vi "Relink Package - LV2020.vi"(8 "error in (no error)":errorcluster) -> (0 "error out":errorcluster, 3 "Folder to Relink out":path=path "C:/Users/JonathanGraesser/Downloads/Delacor QMH")   [LabVIEW 2020]
uses:
  3b4289d2-bfe5-4dee-b35d-c917e2b2519d.vi
  44c3ad98-b52a-4573-a8f5-4ecf539941a0.vi
  7ce98f71-275c-4c1e-b900-7d867c156dbc.vi
  c2568c13-bb09-496e-a5a3-529df0c50f32.vi
panel:
  out "report log out":string[](array[string])
  out "Done":bool
  out "all lv items":path[](array[path])
  in  "Folder to relink":string
  out "Saved Items out":T1(array[cluster])
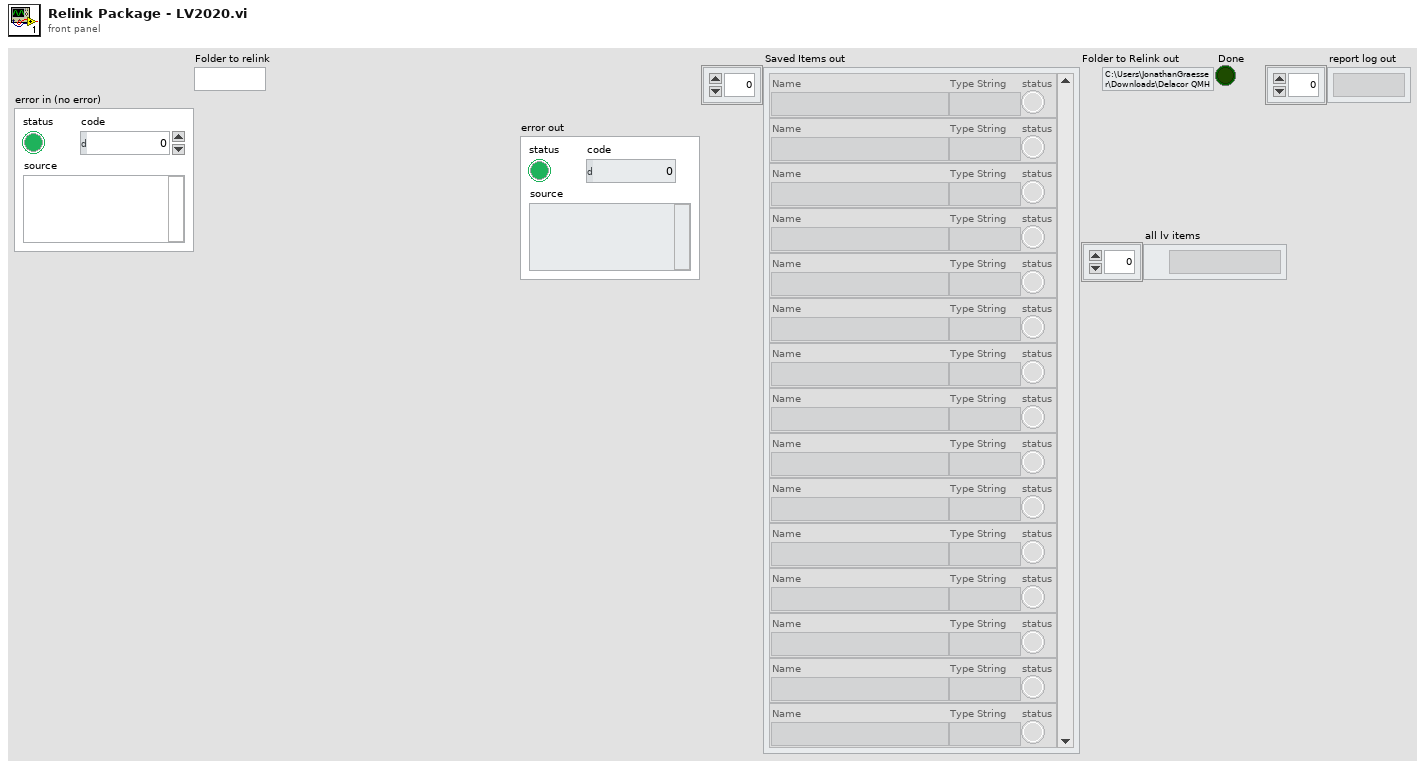
[diagram p1: front panel]
types:
  T1 = cluster{"Name":string, "Type String":string, "status":bool}[]
  T2 = cluster{"Name":string, "Type String":string, "status":bool}
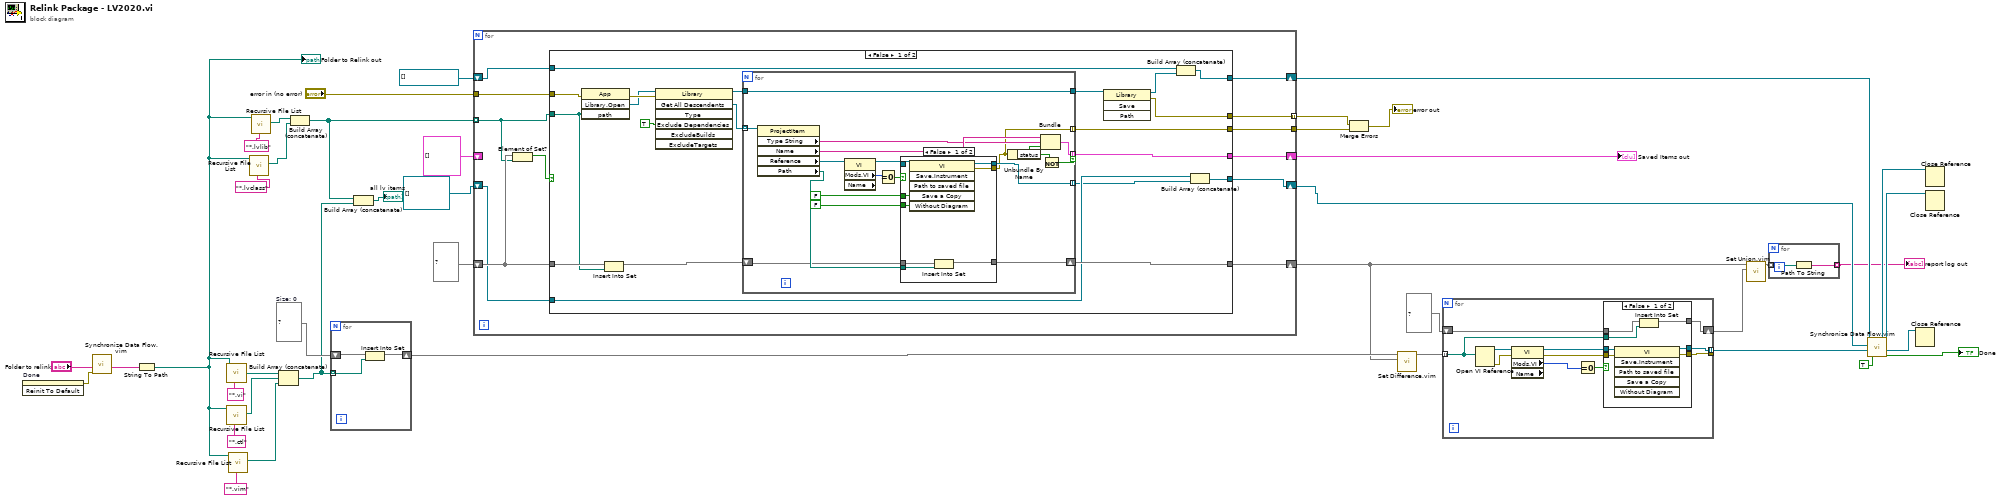
[diagram p0: block diagram]
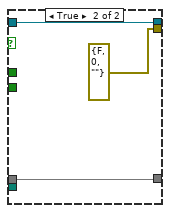
[diagram p2: hidden frame]
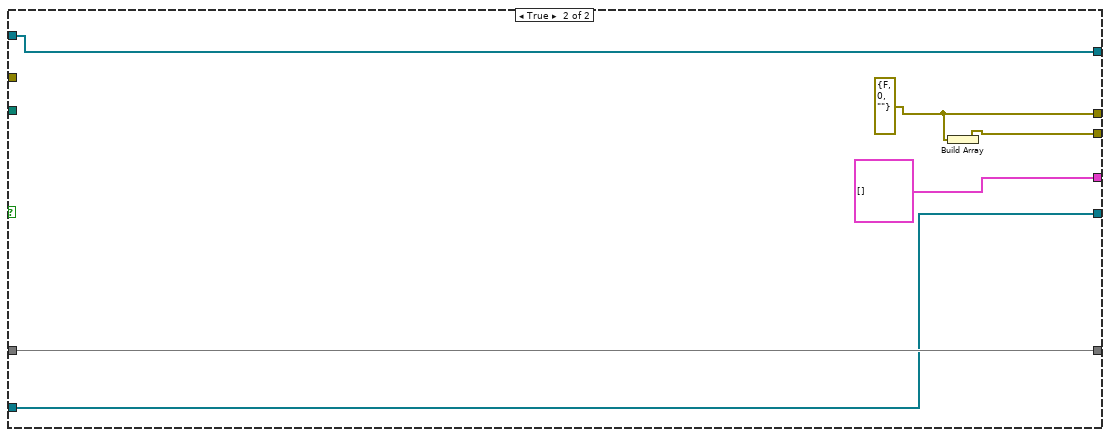
[diagram p3: hidden frame]
diagram:
  w39 = set{path} {}  # Size: 0
  n1 = invoke on="Done" class="Bool (strict)" method="Reinit To Default"() -> (error out=w8:errorcluster)  [unwired: 3 in, 2 out]
  n2 = call "Synchronize Data Flow.vim"("input 4"=w8, "input 3"="Folder to relink") -> ("output 3"=w9:string)  [unwired: 2 in, 3 out]
  n3 = String To Path(string=w9) -> (path=w26:path)
  "Folder to Relink out" <- w26
  n4 = call <vilib>:"Recursive File List.vi"("pattern"="*.vi", "Folder Path"=w26) -> ("All Files in Dir"=w40:path[])  [unwired: 5 in, 4 out]
  n5 = call <vilib>:"Recursive File List.vi"("pattern"="*.ctl", "Folder Path"=w26) -> ("All Files in Dir"=w35:path[])  [unwired: 5 in, 4 out]
  n6 = call <vilib>:"Recursive File List.vi"("pattern"="*.vim", "Folder Path"=w26) -> ("All Files in Dir"=w34:path[])  [unwired: 5 in, 4 out]
  n7 = call <vilib>:"Recursive File List.vi"("pattern"="*.lvclass", "Folder Path"=w26) -> ("All Files in Dir"=w30:path[])  [unwired: 5 in, 4 out]
  n8 = call <vilib>:"Recursive File List.vi"("pattern"="*.lvlib", "Folder Path"=w26) -> ("All Files in Dir"=w31:path[])  [unwired: 5 in, 4 out]
  n9 = Build Array (concatenate)(w40, w35, w34) -> (w13:path[])
  n10 = Build Array (concatenate)(w31, w30) -> (w1:path[])
  n11 = for {
    shift-right: [w44] -> w28
    shift-left: w39 -> [w43]
    tunnel: w13 -> [w45] mode=indexing
    n12 = Insert Into Set(10:w45, 11:w43) -> (3:w44:set{path})  [unwired: 1 out]
  }
  n13 = Build Array (concatenate)(w1, w13) -> (→"all lv items":path[])
  n14 = for {
    shift-right: [w56] -> w3
    shift-left: set{path} {} ("set in") -> [w55]
    tunnel: w1 -> [w54] mode=indexing
    tunnel: "error in (no error)" -> [w52]
    tunnel: [w51] -> w25
    tunnel: [w50] -> w23 mode=indexing
    shift-right: [w48] -> w14
    shift-left: refnum<vi>[] [] ("Open Library") -> [w49]
    shift-right: [w57] -> w42
    shift-left: T1 [] -> [_]
    shift-right: [w46] -> w17
    shift-left: refnum<vi>[] [] -> [w47]
    n15 = Element of Set?(10:w54, 11:w55) -> (3:w53:bool)
    n16 = case shown="False" w53 {
      tunnel: [w73 T1 []] -> w57
      tunnel: [w69 w112] -> w56
      tunnel: w55 -> [w68 w112]
      tunnel: w54 -> [w67 _]
      tunnel: w52 -> [w66 _]
      tunnel: [w58 w107] -> w51
      tunnel: [w65 w108] -> w50
      tunnel: w49 -> [w64 w110]
      tunnel: [w62 w110] -> w48
      tunnel: w47 -> [w61 w109]
      tunnel: [w59 w109] -> w46
      frame False {
        n17 = invoke class="App" method="Library.Open"(error in=w66, "path"=w67) -> (error out=w77:errorcluster, "Open Library"=w76:refnum<vi>)  [unwired: 2 in, 2 out]
        n18 = Insert Into Set(10:w67, 11:w68) -> (3:w70:set{path})  [unwired: 1 out]
        n19 = invoke class="Library" method="Get All Descendents"(reference=w76, error in=w77, "Exclude Dependencies"=TRUE ("ExcludeDependencies")) -> (reference out=w71:refnum<vi>, "All Descendents"=w75:refnum<vi>[])  [unwired: 4 in, 5 out]
        n20 = for {
          tunnel: w75 -> [w95] mode=indexing
          tunnel: [w92] -> w73 mode=indexing if=w88
          tunnel: [w87] -> w72
          tunnel: w71 -> [w87]
          shift-right: [w85] -> w69
          shift-left: w70 -> [w84]
          tunnel: [w83] -> w60 mode=indexing
          tunnel: [w82] -> w58 mode=indexing
          n21 = property class="ProjectItem"(reference=w95) -> ("Type String"=w93:string, "Name"=w94:string, "Reference"=w81:refnum<vi>, "Path"=w86:path)  [unwired: 1 in, 2 out]
          n22 = property class="VI" props=["Mods.VI", "Name"](reference=w81) -> (reference out=w80:refnum<vi>, "Mods.VI"=w79:u64)  [unwired: 1 in, 2 out]
          n23 = Equal To 0?(x=w79) -> (x = 0?=w78:bool)
          n24 = case shown="False" w78 {
            tunnel: FALSE ("Save a Copy") -> [w103 _]
            tunnel: FALSE ("Without Diagram") -> [w102 _]
            tunnel: w86 -> [w101 _]
            tunnel: [w100 w104] -> w85
            tunnel: w84 -> [w99 w104]
            tunnel: [w98 w106] -> w83
            tunnel: [w97 errorcluster {"status"=FALSE, "code"=0, "source"=""} ("error out")] -> w82
            tunnel: w80 -> [w96 w106]
            frame False {
              n25 = invoke class="VI" method="Save.Instrument"(reference=w96, "Save a Copy"=w103, "Without Diagram"=w102) -> (reference out=w98:refnum<vi>, error out=w97:errorcluster)  [unwired: 3 in, 4 out]
              n26 = Insert Into Set(10:w101, 11:w99) -> (3:w100:set{path})  [unwired: 1 out]
            }
            frame True {
            }
          }
          n27 = Unbundle By Name(w82) -> ("status"=w89:bool)
          n28 = Bundle("Name"=w94, "Type String"=w93, "status"=w89) -> (w92:T2)  [unwired: 1 in]
          n29 = Not(x=w89) -> (.not. x?=w88:bool)
        }
        n30 = invoke class="Library" method="Save"(reference=w72) -> (reference out=w63:refnum<vi>, error out=w65:errorcluster)  [unwired: 3 in, 2 out]
        n31 = Build Array (concatenate)(w64, w63) -> (w62:refnum<vi>[])
        n32 = Build Array (concatenate)(w61, w60) -> (w59:refnum<vi>[])
      }
      frame True {
        w108 = errorcluster {"status"=FALSE, "code"=0, "source"=""} ("error out")
        n33 = Build Array(w108) -> (w107:errorcluster[])
      }
    }
  }
  "Saved Items out" <- w42
  n34 = Merge Errors(w23, w25) -> (→"error out":errorcluster)
  n35 = call "Set Difference.vim"("set 2"=w3, "set 1"=w28) -> ("difference"=w5:set{path})  [unwired: 9 in]
  n36 = for {
    tunnel: w5 -> [w114] mode=indexing
    tunnel: [w117] -> _
    tunnel: [w116] -> w19 mode=indexing
    shift-right: [w113] -> w2
    shift-left: set{path} {} ("difference") -> [w115]
    n37 = Open VI Reference(vi path=w114) -> (vi reference=w123:refnum<vi>, error out=w122:errorcluster)  [unwired: 5 in]
    n38 = property class="VI" props=["Mods.VI", "Name"](reference=w123, error in=w122) -> (reference out=w121:refnum<vi>, error out=w120:errorcluster, "Mods.VI"=w118:u64)  [unwired: 1 out]
    n39 = Equal To 0?(x=w118) -> (x = 0?=w119:bool)
    n40 = case shown="False" w119 {
      tunnel: w121 -> [w130 w133]
      tunnel: w120 -> [w129 w132]
      tunnel: [w128 w133] -> w116
      tunnel: [w127 w132] -> w117
      tunnel: w115 -> [w126 w131]
      tunnel: w114 -> [w125 _]
      tunnel: [w124 w131] -> w113
      frame False {
        n41 = invoke class="VI" method="Save.Instrument"(reference=w130, error in=w129) -> (reference out=w128:refnum<vi>, error out=w127:errorcluster)  [unwired: 4 in, 4 out]
        n42 = Insert Into Set(10:w125, 11:w126) -> (3:w124:set{path})  [unwired: 1 out]
      }
      frame True {
      }
    }
  }
  n43 = call "Set Union.vim"("set 2"=w2, "set 1"=w3) -> ("union"=w7:set{path})  [unwired: 9 in]
  n44 = for {
    tunnel: [w134] -> w6 mode=indexing
    tunnel: w7 -> [w135] mode=indexing
    n45 = Path To String(path=w135) -> (string=w134:string)
  }
  "report log out" <- w6
  n46 = call "Synchronize Data Flow.vim"("input 4"=TRUE, "input 3"=w19, "input 2"=w17, "input 1"=w14) -> ("output 4"=→"Done":bool, "output 3"=w18:refnum<vi>[], "output 2"=w16:refnum<vi>[], "output 1"=w15:refnum<vi>[])
  n47 = Close Reference(reference=w18) -> ()  [unwired: 1 in, 1 out]
  n48 = Close Reference(reference=w15) -> ()  [unwired: 1 in, 1 out]
  n49 = Close Reference(reference=w16) -> ()  [unwired: 1 in, 1 out]
